vi "FTW-Regex-Construct.vi"(5 "Regular Expression":string, 11 "error in":errorcluster) -> (4 "Regex":refnum<data-value>, 15 "error out":errorcluster)   [LabVIEW 2015]
uses:
  core/FTW-Regex-Core-Structure.ctl
panel:
  # "Inputs"
  # "Outputs"
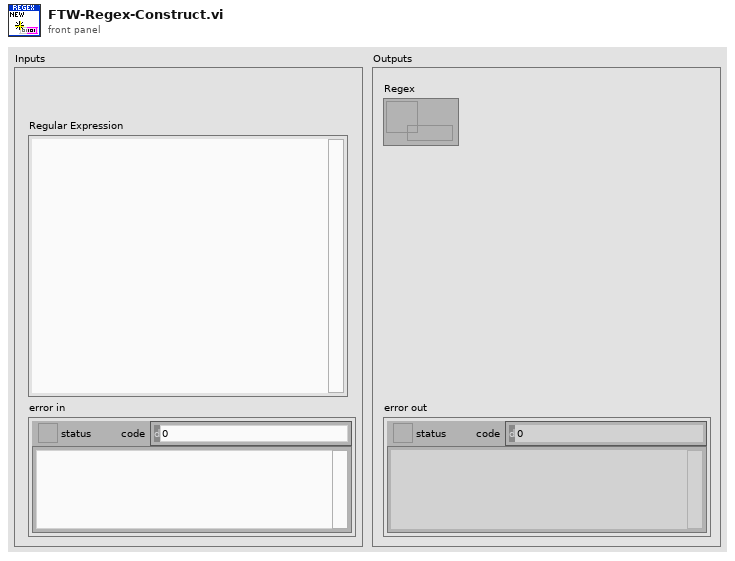
[diagram p1: front panel]
types:
  T1 = typedef "FTW-Regex-Core-Structure.ctl" = cluster{"Compiled Regex":u64}
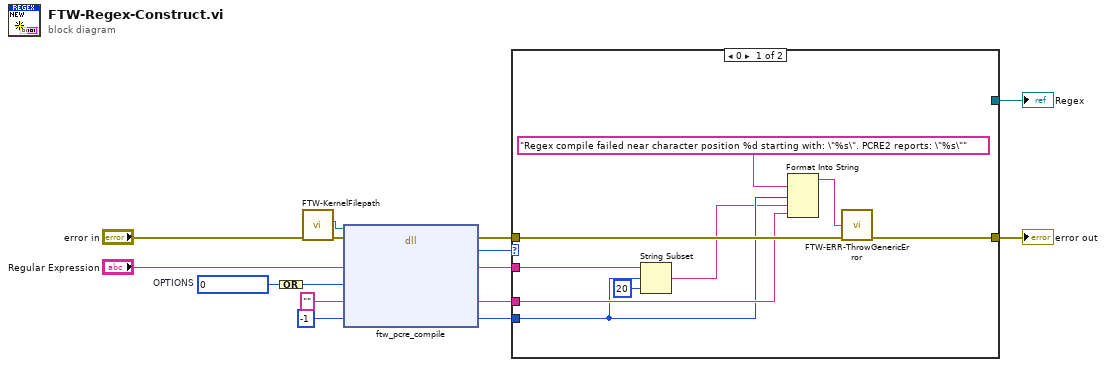
[diagram p0: block diagram]
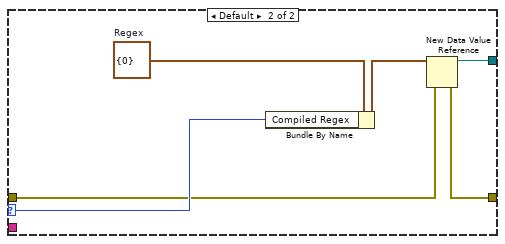
[diagram p2: hidden frame]
diagram:
  w13 = u32 0  # OPTIONS
  n1 = Compound Arithmetic op=OR(w13) -> (w14:u32)
  n2 = call "FTW-KernelFilepath.vi"("error in"="error in") -> ("error out"=w2:errorcluster, "Library Filepath"=w1:path)  [unwired: 8 in, 1 out]
  n3 = dll-call lib="?" fn="ftw_pcre_compile"(path in=w1, error in=w2, "Pattern"="Regular Expression", "Options"=w14, "Error String"="", "Error Offset in Pattern"=-1) -> (error out=w9:errorcluster, "Compiled Regex"=w11:u64, "Pattern"=w4:string, "Error String"=w7:string, "Error Offset in Pattern"=w5:i32)  [unwired: 2 in, 1 out]
  n4 = case shown="0" w11 {
    selector: w11 -> [_ w30]
    tunnel: [_ w27] -> w10
    tunnel: w9 -> [w24 w26]
    tunnel: [w23 w25] -> w8
    tunnel: w7 -> [w20 _]
    tunnel: w5 -> [w18 _]
    tunnel: w4 -> [w19 _]
    frame 0 {
      n5 = String Subset(string=w19, offset (0)=w18, length (rest)=20 ("length (rest)")) -> (substring=w16:string)
      n6 = Format Into String(format string="Regex compile failed near character position %d starting with: \"%s\". PCRE2 reports: \"%s\"", w18, w16, w20) -> (resulting string=w22:string)  [unwired: 2 in, 1 out]
      n7 = call "FTW-ERR-ThrowGenericError.vi"("Error Message"=w22, "error in"=w24) -> ("error out"=w23:errorcluster)  [unwired: 13 in]
    }
    frame Default {
      w29 = T1 {"Compiled Regex"=0}  # Regex
      n8 = Bundle By Name(cluster=w29, "Compiled Regex"=w30) -> (w28:T1)
      n9 = New Data Value Reference(data value=w28, error in=w26) -> (data value reference=w27:refnum<data-value>, error out=w25:errorcluster)
    }
  }
  "error out" <- w8
  "Regex" <- w10
